vi "ScratchOrNew.vi"(9 "Test btn":bool, 11 "Template":string) -> (2 "Success":bool, 3 "Settings Out":T1={"Name of test"="", "Date"=timestamp(0 s since 1904-01-01), "Location"="", "Template"="", "Soundcard"="", "resolution"=0, "Sampling rate"=0, "Ch1 Gain "=0.0, "Ch2 Gain"=0.0, "Sample time (s)"=0.0, "Pre-trigger (s)"=0.0, "Hammer Threshold"=0.0, "Positions"=0, "Taps/Position"=0, "Set Names"="", "Freq resolution"=0.0, "Hammer cutoff"=0.0, "Mic cutoff"=0.0, "Double bounce "=0.0, "Hammer Cal"=0.0, "dB Offset"=0.0, "Accel Cal"=0.0, "Vibrometer Cal"=0.0, "Mic Cal"=0.0, "Output"=0, "Voltage Cal"=0.0, "Vibrometer Port"="", "Range"=0, "High Pass"=0, "Bandwidth"=0, "X Range"=[], "Y Range"=[], "dB Spread"=0.0, "Trigger"=0, "Ch_1"=0, "Ch_2"=0, "flip?"=FALSE, "60Hz"=FALSE, "Time offset"=0.0, "Piezo Cal"=1.0, "Default Notes"="", "Tom"=FALSE} {"Ch_2" min=1 step=1; "Ch_1" min=1 max=100 step=1; "Trigger" items=["Hammer (force)", "Self-tap", "Spacebar"]; "Bandwidth" items=["1 kHz"=1, "5 kHz"=5, "10 kHz"=10, "25 kHz"=25, "50 kHz"=50, "100 kHz"=100]; "High Pass" items=["Off", "13 Hz", "104 Hz"]; "Range" items=["10 mm/s"=1, "20 mm/s"=2, "50 mm/s"=5, "100 mm/s"=10, "200 mm/s"=20, "500 mm/s"=50, "1 m/s"=100, "2 m/s"=200]; "Output" items=["Accelerometer", "Speed (from acceleration)", "Microphone", "Vibrometer", "Piezo"]; "Voltage Cal" format="%#_13g"; "Ch2 Gain" format="%#_13g"; "Ch1 Gain" format="%#_13g"; "Double bounce" min=0.0; "Mic cutoff" min=0.0 format="%#_4g"; "Hammer cutoff" min=0.0 format="%#_4g"; "Freq resolution" min=0.0; "Pre-trigger (s)" format="%#_13g"; "Date" format="%<%H:%M\n%d/%m/%y>T"; "resolution" items=["16 bit"=16, "24 bit"=24, "32 bit"=32]; "Sampling rate" items=["22050 samp/s"=22050, "44100 samp/s"=44100, "48000 samp/s"=48000]})   [LabVIEW 2022 SP3]
uses:
  PreferencesControl.ctl
  Mic/Mic_Global.vi
panel:
  in  "device:":u16(ring) items=["BuerginBase Microphone", "485B39 200083408035100798118210422", "MacBook Pro Microphone", "Microsoft Teams Audio"]
  # "Hz"
  # "dB"
  # "dB"
  # "sec"
  # "sec"
  # "mV/Pa"
  # "mV/m/s2"
  # "mV/mm/s"
  # "V/N"
  # "sec"
  # "sec"
  # "mV/N"
  # "a.u."
  # "a.u."
  # "sec"
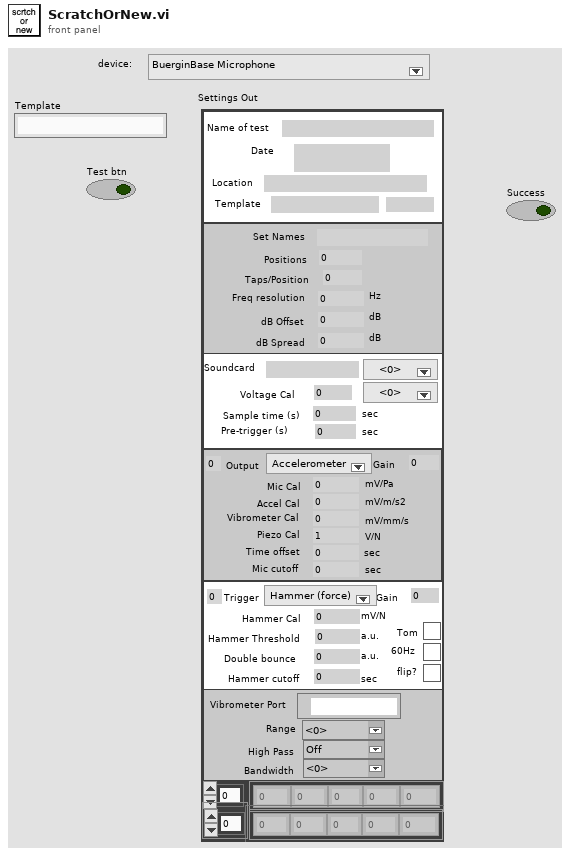
[diagram p1: front panel]
types:
  T1 = typedef "PreferencesControl.ctl" = cluster{"Name of test":string, "Date":timestamp, "Location":string, "Template":string, "Soundcard":string, "resolution":u16, "Sampling rate":u16, "Ch1 Gain ":dbl, "Ch2 Gain":dbl, "Sample time (s)":dbl, "Pre-trigger (s)":dbl, "Hammer Threshold":dbl, "Positions":i16, "Taps/Position":i16, "Set Names":string, "Freq resolution":dbl, "Hammer cutoff":dbl, "Mic cutoff":dbl, "Double bounce ":dbl, "Hammer Cal":dbl, "dB Offset":dbl, "Accel Cal":dbl, "Vibrometer Cal":dbl, "Mic Cal":dbl, "Output":u16, "Voltage Cal":dbl, "Vibrometer Port":refnum<visa-resource-name>, "Range":u16, "High Pass":u16, "Bandwidth":u16, "X Range":cluster{"Minimum":dbl, "Maximum":dbl, "Increment":dbl, "Minor Increment":dbl, "Start":dbl}[], "Y Range":cluster{"Minimum":dbl, "Maximum":dbl, "Increment":dbl, "Minor Increment":dbl, "Start":dbl}[], "dB Spread":dbl, "Trigger":u16, "Ch_1":u8, "Ch_2":u8, "flip?":bool, "60Hz":bool, "Time offset":dbl, "Piezo Cal":dbl, "Default Notes":string, "Tom":bool}
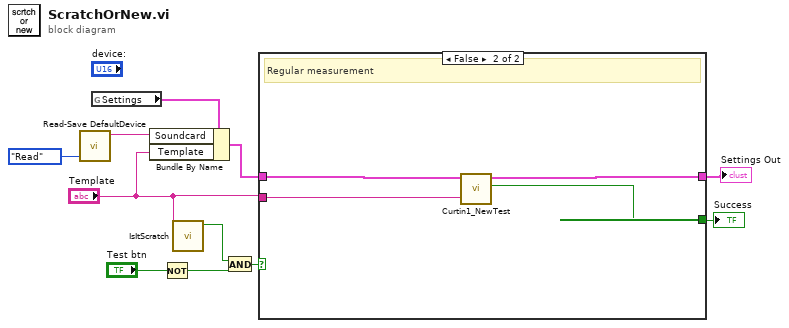
[diagram p0: block diagram]
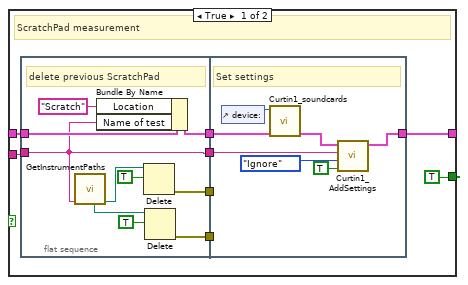
[diagram p2: hidden frame]
diagram:
  n1 = call "Read-Save DefaultDevice.vi"("Task"=enum16{"Save", "Read"}."Read") -> ("Soundcard Out"=w3:string)  [unwired: 9 in, 1 out]
  n2 = global read "Mic_Global.vi" "Settings"() -> (w4:T1)
  n3 = Bundle By Name(cluster=w4, "Soundcard"=w3, "Template"="Template") -> (w2:T1)
  n4 = Not(x="Test btn") -> (.not. x?=w8:bool)
  n5 = call "IsItScratch.vi"("Template"="Template") -> ("ScratchPad?"=w10:bool)  [unwired: 10 in]
  n6 = And(x=w10, y=w8) -> (x .and. y?=w7:bool)
  n7 = case shown="False" w7 {
    tunnel: "Template" -> [w19 w38]
    tunnel: [w18 w40] -> w6
    tunnel: [TRUE ("Date?") w39] -> w11
    tunnel: w2 -> [w13 w37]
    frame True {
      # "ScratchPad measurement"
      n8 = flat-sequence {
        tunnel: w19 -> [w21]
        tunnel: [w21] -> w16
        tunnel: [w25] -> w15
        tunnel: [w24] -> w14
        tunnel: w13 -> [w23]
        tunnel: [w22] -> w12
        tunnel: w16 -> [w34]
        tunnel: [w35] -> w18
        tunnel: w15 -> [_]
        tunnel: w14 -> [_]
        tunnel: w12 -> [w32]
        frame #0 {
          # "delete previous ScratchPad"
          n9 = call "GetInstrumentPaths.vi"("Instrument"=w21) -> ("Path To Raw Folder"=w28:path, "Path To TRF Folder"=w29:path)  [unwired: 6 in, 3 out]
          n10 = Bundle By Name(cluster=w23, "Location"="Scratch", "Name of test"=w21) -> (w22:T1)
          n11 = Delete(path (use dialog)=w28, entire hierarchy (F)=TRUE) -> (error out=w24:errorcluster)  [unwired: 3 in, 2 out]
          n12 = Delete(path (use dialog)=w29, entire hierarchy (F)=TRUE) -> (error out=w25:errorcluster)  [unwired: 3 in, 2 out]
        }
        frame #1 {
          # "Set settings"
          n13 = control-ref of="device:"() -> (w30:refnum<vi>)
          n14 = call "Curtin1_soundcards.vi"("Settings In"=w32, "device:"=w30) -> ("Settings Out"=w31:T1)  [unwired: 8 in, 1 out]
          n15 = call "Curtin1_AddSettings.vi"("Date?"=TRUE, "Check?"=enum16{"Ignore", "Check", "Replace"}."Ignore", "Template"=w34, "Settings in"=w31) -> ("Settings Out"=w35:T1)  [unwired: 6 in, 1 out]
        }
      }
    }
    frame False {
      # "Regular measurement"
      n16 = call "Curtin1_NewTest.vi"("Template name"=w38, "Settings"=w37) -> ("Success"=w39:bool, "Settings Out"=w40:T1)  [unwired: 8 in]
    }
  }
  "Settings Out" <- w6
  "Success" <- w11
